vi "Edit Value.vi"(6 "Action":T1, 8 "error in (no error)":errorcluster, 10 "New Val":dbl, 11 "Sample in":refnum<class "Sample.lvclass">) -> (0 "error out":errorcluster, 3 "Sample out":refnum<class "Sample.lvclass">)   [LabVIEW 2020, in "Metrics.lvlib" / "Sample.lvclass"]
uses:
  Sample.lvclass
  Edit Action.ctl
  Sample.lvclass/Sample.ctl
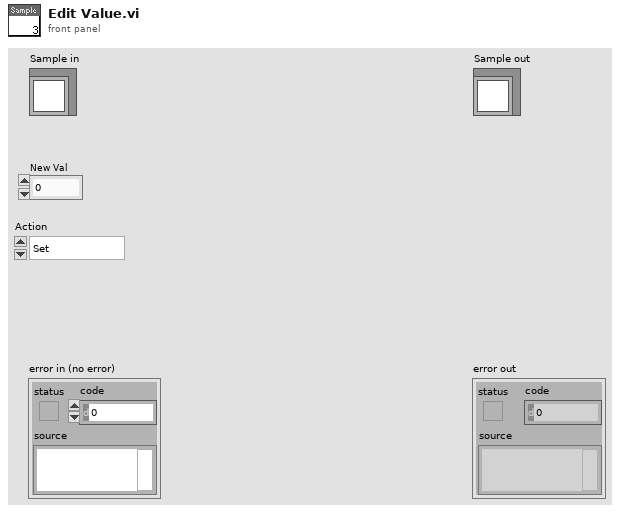
[diagram p1: front panel]
types:
  T1 = typedef "Metrics.lvlib/Sample.lvclass/Edit Action.ctl" = enum16{"Set", "Increment"}
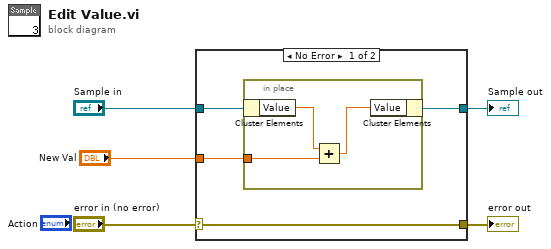
[diagram p0: block diagram]
diagram:
  n1 = case shown="No Error" "error in (no error)" {
    selector: "error in (no error)" -> [w9 w14]
    tunnel: [w9 w14] -> w4
    tunnel: [w6 w13] -> w2
    tunnel: "Sample in" -> [w8 w13]
    tunnel: "New Val" -> [w7 _]
    frame No Error {
      n2 = in-place {
        in-place-border: w7 -> [w11]
        n3 = in-place-cluster #1(w8) -> ("Value"=w12:dbl)
        n4 = Add(x=w12, y=w11) -> (x+y=w10:dbl)
        n5 = in-place-cluster #1("Value"=w10) -> (w6:refnum<class "Sample.lvclass">)
      }
    }
    frame Error {
    }
  }
  "error out" <- w4
  "Sample out" <- w2
